vi "Ds18b20 ID.vi"() -> ()   [LabVIEW 2014, in "QwaveSys RPi Training Library.lvlib"]
uses:
  <vilib>/Q-Wave Systems/QwaveSys RPi Training Package (Demo)/Addons/QwaveSys RPi Training Library.lvlib
panel:
  out "Ds18b20 ID":string
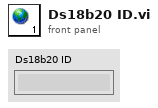
[diagram p1: front panel]
diagram:
